vi "Set Master Bitfile.vi"(7 "MulticolumnListbox in":refnum<vi>, 8 "error in (no error)":errorcluster, 9 "listbox text":string[][](array[string]), 10 "Selected Value":i32, 11 "Item Ref in":T1 format="%.0x") -> (0 "error out":errorcluster, 3 "Item Ref out":T1 format="%.0x")   [LabVIEW 2015, in "Engine Simulation Toolkit System Explorer.lvlib"]
uses:
  Engine Simulation Toolkit System Explorer.lvlib
  <vilib>/NI Veristand/Custom Device API/Custom Device Item Ref.ctl
  Shared/Properties.vi
  <vilib>/NI Veristand/Custom Device API/Set Item Property (String).vi
  Shared/Engine Simulation Toolkit Shared.lvlib
  <vilib>/NI Veristand/Custom Device API/Custom Device API.lvlib
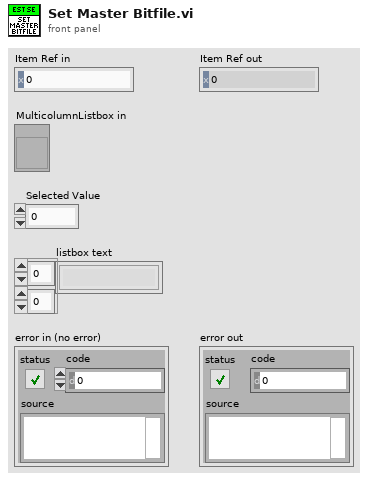
[diagram p1: front panel]
types:
  T1 = typedef "Custom Device API.lvlib/Custom Device Item Ref.ctl" = u64
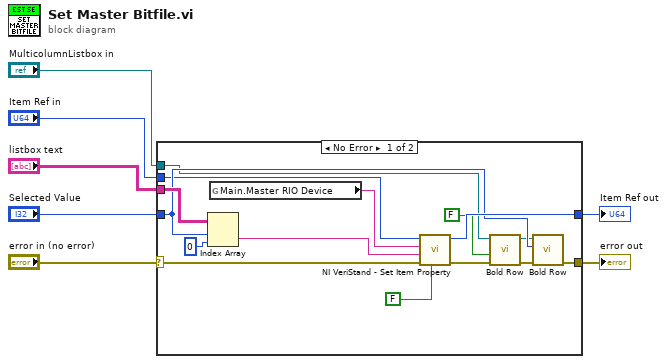
[diagram p0: block diagram]
diagram:
  n1 = case shown="No Error" "error in (no error)" {
    selector: "error in (no error)" -> [w12 w24]
    tunnel: "listbox text" -> [w22 _]
    tunnel: [w21 w23] -> w6
    tunnel: [w20 w24] -> w5
    tunnel: "Selected Value" -> [w18 w23]
    tunnel: "MulticolumnListbox in" -> [w14 _]
    tunnel: "Item Ref in" -> [w11 _]
    frame No Error {
      n2 = Index Array(array=w22, index (row)=w18, index (col)=0 ("disabled index (col)")) -> (element=w10:string)
      n3 = global read "Properties.vi" "Main.Master RIO Device"() -> (w9:string)
      n4 = call-poly <vilib>:"NI VeriStand - Set Item Property.vi"("Binary String (T)"=FALSE, "error in (no error)"=w12, "Value"=w10, "Property Name"=w9, "Item Ref in"=w11) -> ("error out"=w13:errorcluster, "Item Ref out"=w21:T1)  [unwired: 4 in, 1 out]
      n5 = call "Bold Row.vi"("error in (no error)"=w13, "Bold? (T)"=FALSE ("Bold?"), "MulticolumnListbox in"=w14) -> ("error out"=w15:errorcluster, "MulticolumnListbox out"=w16:refnum<vi>)  [unwired: 7 in]
      n6 = call "Bold Row.vi"("error in (no error)"=w15, "Row (-2 : all)"=w18, "MulticolumnListbox in"=w16) -> ("error out"=w20:errorcluster)  [unwired: 7 in, 1 out]
    }
    frame Error {
    }
  }
  "Item Ref out" <- w6
  "error out" <- w5
